vi "Deinitialize.vi"(11 "Modbus master in":refnum<class "Modbus Master.lvclass">) -> (0 "error out":errorcluster)   [LabVIEW 2023, in "RS485.lvlib"]
uses:
  RS485.lvlib
  <vilib>/NI/Modbus Library/API/Master/Modbus Master.lvclass
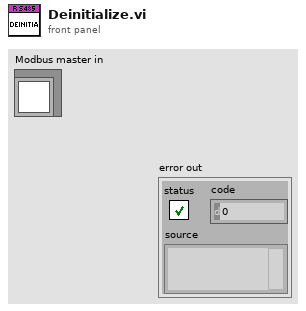
[diagram p1: front panel]
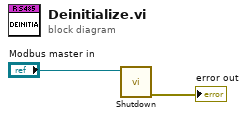
[diagram p0: block diagram]
diagram:
  n1 = call-dynamic "Shutdown.vi"("Modbus master in"="Modbus master in") -> ("error out"=→"error out":errorcluster)  [unwired: 10 in]
